vi "4 Opérations.vi"() -> ()   [LabVIEW 2018]
panel:
  out "X*Y":dbl
  out "X/Y":dbl
  out "X-Y":dbl
  out "X+Y":dbl
  in  "Y":dbl min=0.0 max=9.0
  in  "X":dbl min=0.0 max=9.0
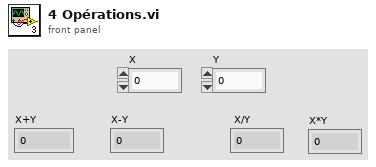
[diagram p1: front panel]
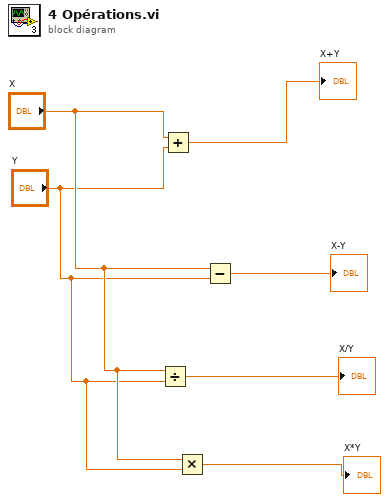
[diagram p0: block diagram]
diagram:
  n1 = Divide(x="X", y="Y") -> (x/y=→"X/Y":dbl)
  n2 = Add(x="X", y="Y") -> (x+y=→"X+Y":dbl)
  n3 = Multiply(x="X", y="Y") -> (x*y=→"X*Y":dbl)
  n4 = Subtract(x="X", y="Y") -> (x-y=→"X-Y":dbl)
